vi "TestInitializeAbstractPolicy_Error.vi"(8 "error in (no error)":errorcluster, 11 "TestCase in":refnum<class "TestSubscriptionPolicy.lvclass">) -> (0 "error out":errorcluster, 3 "TestCase out":refnum<class "TestSubscriptionPolicy.lvclass">)   [LabVIEW 2020, in "TestSubscriptionPolicy.lvclass"]
uses:
  TestSubscriptionPolicy.lvclass
  TestSubscriptionPolicy.lvclass/TestSubscriptionPolicy.ctl
  Source/IMediator/ISubscriptionPolicy/ISubscriptionPolicy.lvclass
  modules/composed-transport/Source/Concrete/QueueTransport/QueueTransport.lvclass
  C:/Git/mva-core/modules/composed-transport/Source/ITransport/ITransport.lvclass
  C:/Git/mva-core/modules/composed-transport/Source/Concrete/QueueTransport/QueueTransport.lvclass
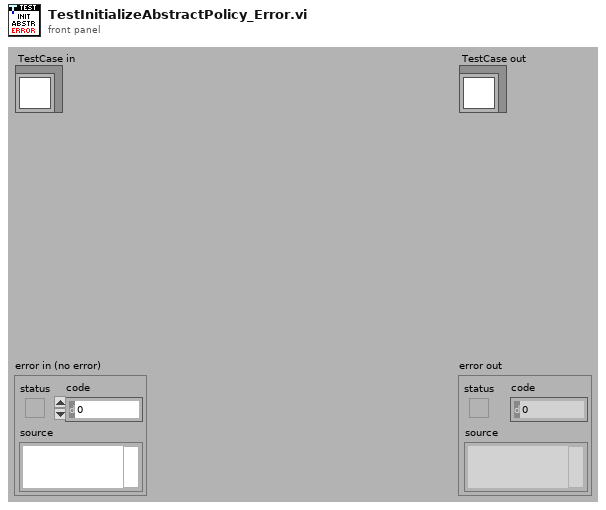
[diagram p1: front panel]
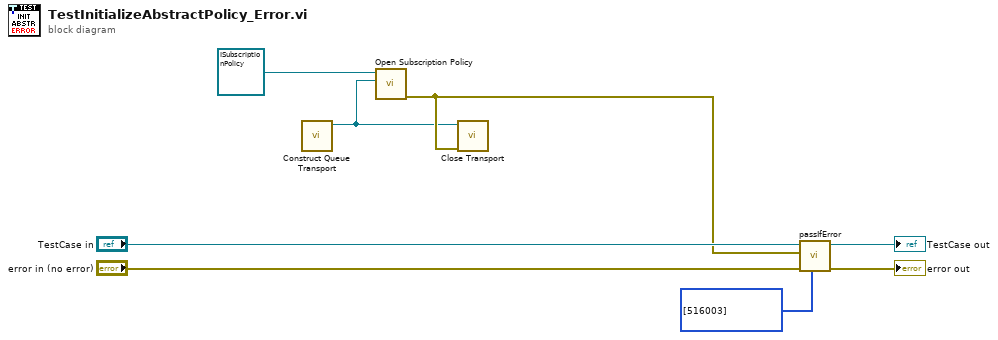
[diagram p0: block diagram]
diagram:
  n1 = call "Construct Queue Transport.vi"() -> ("QueueTransport"=w2:refnum<class "QueueTransport.lvclass">)  [unwired: 10 in, 1 out]
  n2 = call "Open Subscription Policy.vi"("Transport"=w2, "SubscriptionPolicy"=refnum<class "ISubscriptionPolicy.lvclass"> refnum ("IMediator.lvlib:ISubscriptionPolicy.lvclass")) -> ("error out"=w3:errorcluster)  [unwired: 8 in, 1 out]
  n3 = call-dynamic "Close Transport.vi"("error in (no error)"=w3, "QueueTransport"=w2) -> ()  [unwired: 9 in, 1 out]
  n4 = call-dynamic "passIfError.vi"("passing error codes (default = any error code)"=i32[] [516003], "error in (no error)"="error in (no error)", "error"=w3, "TestCase in"="TestCase in") -> ("error out"=→"error out":errorcluster, "TestCase out"=→"TestCase out":refnum<class "TestSubscriptionPolicy.lvclass">)  [unwired: 6 in]
